vi "Log Data.vi"() -> ()   [LabVIEW 2013]
panel:
  in  "Spike Kicking":bool
  in  "Shooter Wheel Speed":dbl
  in  "Wanted RPM":dbl
  in  "Shooter Pot Value":dbl
  in  "RPM":dbl
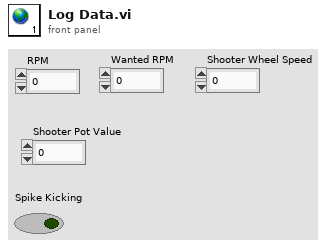
[diagram p1: front panel]
diagram:
